vi "UI.ManagePropertiesView.vi"(8 "error in (no error)":errorcluster, 10 "NewVal":T4, 11 "State Variables":T1={"Aliases.All"=[], "Aliases.Outputs"=[], "UI.Sequence#ofColumns"=0, "SysDef.Path"=path "", "UI.SequenceRef"=refnum, "UI.StepInformationRef"=refnum, "UI.AbortRef"=refnum, "UI.GraphRef"=refnum, "UI.ViewRef"=refnum, "UI.IterationsRef"=refnum, "UI.IterationInformationRef"=refnum, "INI.Settings"={"Build Location"=path "C:/Simple Sequence Editor/SequenceRepo", "LoggingLocation"=path ""}}) -> (0 "error out":errorcluster)   [LabVIEW 2013, in "Simple Sequence Tools - Editor.lvlib"]
uses:
  Simple Sequence Tools - Editor.lvlib
  Types/UI.PropertiesTypes.ctl
  Types/StateVariables.ctl
  Shared/Types/ChannelProperties.ctl
  Shared/Types/INI.Settings
  Shared/Simple Sequence Tools - Shared.lvlib
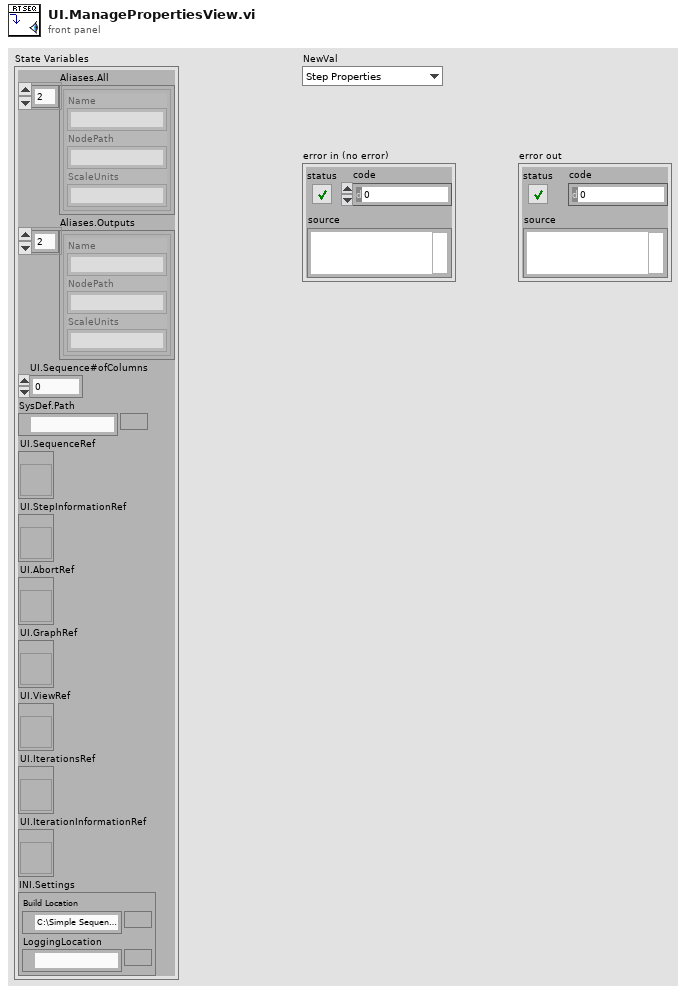
[diagram p1: front panel]
types:
  T1 = typedef "Simple Sequence Tools - Editor.lvlib/StateVariables.ctl" = cluster{"Aliases.All":T2[], "Aliases.Outputs":T2[], "UI.Sequence#ofColumns":i32, "SysDef.Path":path, "UI.SequenceRef":refnum<vi>, "UI.StepInformationRef":refnum<vi>, "UI.AbortRef":refnum<vi>, "UI.GraphRef":refnum<vi>, "UI.ViewRef":refnum<vi>, "UI.IterationsRef":refnum<vi>, "UI.IterationInformationRef":refnum<vi>, "INI.Settings":T3}
  T2 = typedef "Simple Sequence Tools - Shared.lvlib/ChannelProperties.ctl" = cluster{"Name":string, "NodePath":string, "ScaleUnits":string}
  T3 = typedef "Simple Sequence Tools - Shared.lvlib/INI.Settings" = cluster{"Build Location":path, "LoggingLocation":path}
  T4 = typedef "Simple Sequence Tools - Editor.lvlib/UI.PropertiesTypes.ctl" = enum8{"Step Properties", "Sequence Properties"}
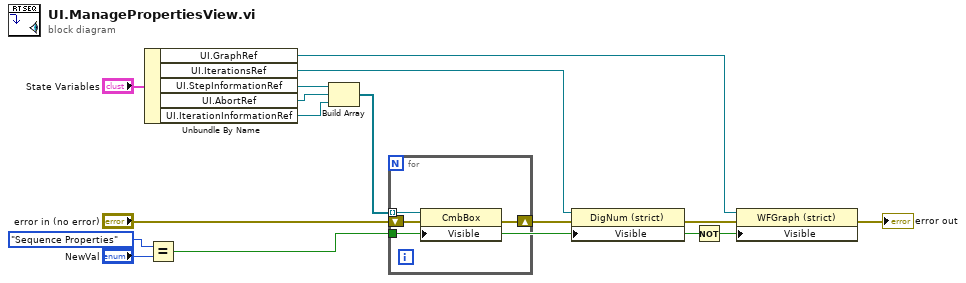
[diagram p0: block diagram]
diagram:
  n1 = Unbundle By Name("State Variables") -> ("UI.GraphRef"=w9:refnum<vi>, "UI.IterationsRef"=w11:refnum<vi>, "UI.StepInformationRef"=w2:refnum<vi>, "UI.AbortRef"=w3:refnum<vi>, "UI.IterationInformationRef"=w15:refnum<vi>)
  n2 = Equal?(x=UI.PropertiesTypes."Sequence Properties" ("View"), y="NewVal") -> (x = y?=w14:bool)
  n3 = Build Array(w2, w3, w15) -> (w4:refnum<vi>[])
  n4 = for {
    tunnel: w4 -> [w19] mode=indexing
    shift-right: [w17] -> w12
    shift-left: "error in (no error)" -> [w18]
    tunnel: w14 -> [w16]
    n5 = property class="CmbBox"(reference=w19, error in=w18, "Visible"=w16) -> (error out=w17:errorcluster)  [unwired: 1 out]
  }
  n6 = property class="DigNum (strict)"(reference=w11, error in=w12, "Visible"=w14) -> (error out=w13:errorcluster)  [unwired: 1 out]
  n7 = Not(x=w14) -> (.not. x?=w10:bool)
  n8 = property class="WFGraph (strict)"(reference=w9, error in=w13, "Visible"=w10) -> (error out=→"error out":errorcluster)  [unwired: 1 out]
